vi "snType(SNXL).vi"(10 "SNXn":string, 11 "SNType":string) -> (3 "show_str_SNwithWholeFormat":string)   [LabVIEW 2011]
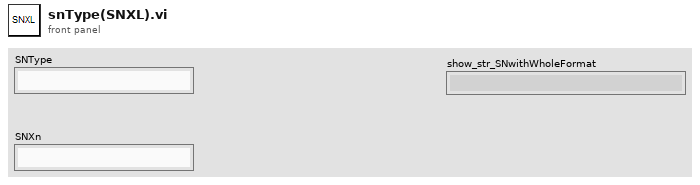
[diagram p1: front panel]
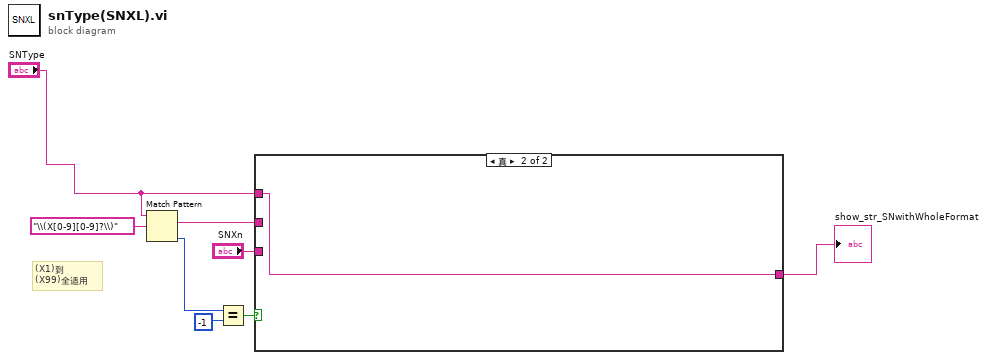
[diagram p0: block diagram]
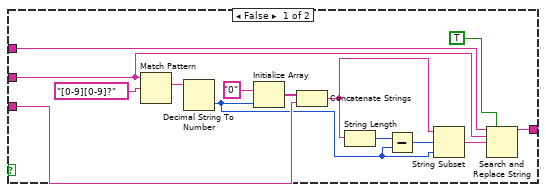
[diagram p2: hidden frame]
diagram:
  # "(X1)到\n(X99)全适用"
  n1 = Match Pattern(string="SNType", regular expression="\\(X[0-9][0-9]?\\)" ("搜索字符串")) -> (match substring=w3:string, offset past match=w7:i32)  [unwired: 1 in, 2 out]
  n2 = Equal?(x=w7, y=-1) -> (x = y?=w5:bool)
  n3 = case shown="真" w5 {
    tunnel: "SNXn" -> [w18 _]
    tunnel: w3 -> [w12 _]
    tunnel: "SNType" -> [w11 w23]
    tunnel: [w9 w23] -> w2
    frame False {
      n4 = Match Pattern(string=w12, regular expression="[0-9][0-9]?" ("正则表达式")) -> (match substring=w21:string)  [unwired: 1 in, 3 out]
      n5 = Decimal String To Number(string=w21) -> (number=w15:i32)  [unwired: 2 in, 1 out]
      n6 = Initialize Array("0", w15) -> (w19:string[])
      n7 = Concatenate Strings(w19, w18) -> (w17:string)
      n8 = String Length(string=w17) -> (length=w16:i32)
      n9 = Subtract(x=w16, y=w15) -> (x-y=w14:i32)
      n10 = String Subset(string=w17, offset (0)=w14, length (rest)=w15) -> (substring=w13:string)
      n11 = Search and Replace String(replace all?=TRUE ("替换全部？(F)"), input string=w11, search string=w12, replace string=w13) -> (result string=w9:string)  [unwired: 4 in, 3 out]
    }
    frame True {
    }
  }
  "show_str_SNwithWholeFormat" <- w2
